vi "Analysis.Result Summaries to Station Result Info_V2.vi"(11 "ResultSum":T2) -> (3 "Pareto Gen Input":T1)   [LabVIEW 2024]
uses:
  Analysis.Result Summary_V2.ctl
  Analysis.Station Fail Paredo Gen Input_V2.ctl
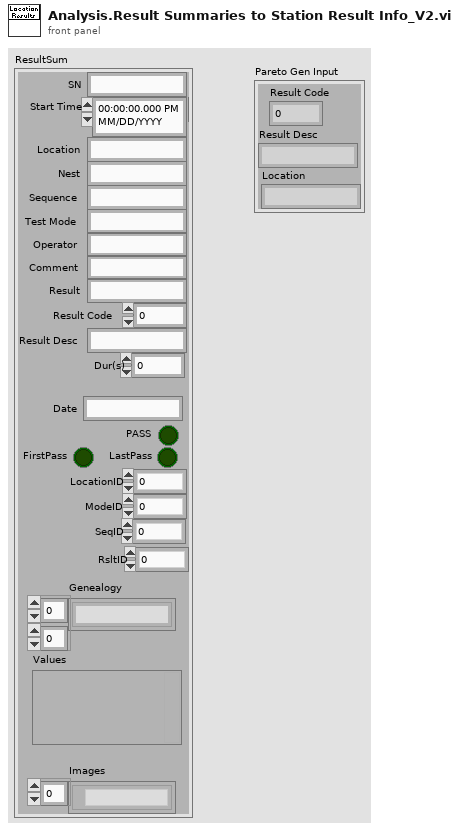
[diagram p1: front panel]
types:
  T1 = typedef "Analysis.Station Fail Paredo Gen Input_V2.ctl" = cluster{"Result Code":i32, "Result Desc":string, "Location":string}
  T2 = typedef "Analysis.Result Summary_V2.ctl" = cluster{"SN":string, "Start Time":timestamp, "Location":string, "Nest":string, "Sequence":string, "Operator":string, "Test Mode":string, "Comment":string, "Result":string, "Result Code":i32, "Result Desc":string, "Date":string, "Dur(s)":dbl, "PASS":bool, "FirstPass":bool, "LastPass":bool, "LocationID":i32, "ModeID":i32, "SeqID":i32, "RsltID":i32, "Genealogy":string[][], "Values":variant, "Images":path[]}
  T3 = cluster{"Result Code":i32, "Result Desc":string, "Location":string}
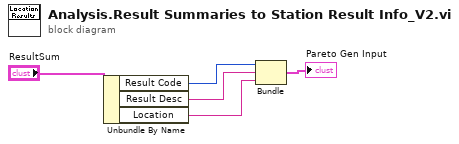
[diagram p0: block diagram]
diagram:
  n1 = Unbundle By Name("ResultSum") -> ("Result Code"=w4:i32, "Result Desc"=w3:string, "Location"=w1:string)
  n2 = Bundle("Result Code"=w4, "Result Desc"=w3, "Location"=w1) -> (→"Pareto Gen Input":T3)  [unwired: 1 in]
